vi "InstrumentInteraction ConfigureMeasurementDigits.vi"(6 "contextId":T1, 8 "error in":errorcluster, 9 "timeout (ms)":i32=-1, 10 "Request Data":T3, 11 "gRPC ID":T1) -> (0 "error out":errorcluster, 2 "Response Data":T2, 3 "gRPC ID out":T1)   [LabVIEW 2020, in "Instrument Interaction Client.lvlib"]
uses:
  Instrument Interaction Client.lvlib
  <vilib>/gRPC/LabVIEW gRPC Library/Shared/grpcId.ctl
  RPC Messages/external_driver_wrapper_ConfigureMeasurementDigitsRequest.ctl
  RPC Messages/external_driver_wrapper_ConfigureMeasurementDigitsResponse.ctl
  RPC Messages/external_driver_wrapper_ConfigureMeasurementDigitsResponse_Flat.ctl
  14035477-4c25-4107-8ed5-d0c4ef420ce5.vi
  <vilib>/gRPC/LabVIEW gRPC Library/Shared/TranslateGrpcError.vi
  <vilib>/gRPC/LabVIEW gRPC Library/Shared/Wait On Occurence.vi
  <vilib>/gRPC/LabVIEW gRPC Library/Server API/Server/Get Server DLL Path.vi
  <vilib>/Utility/error.llb/Error Cluster From Error Code.vi
  <vilib>/Utility/error.llb/Simple Error Handler.vi
  <vilib>/gRPC/LabVIEW gRPC Library/grpc-lvsupport-release.lvlib
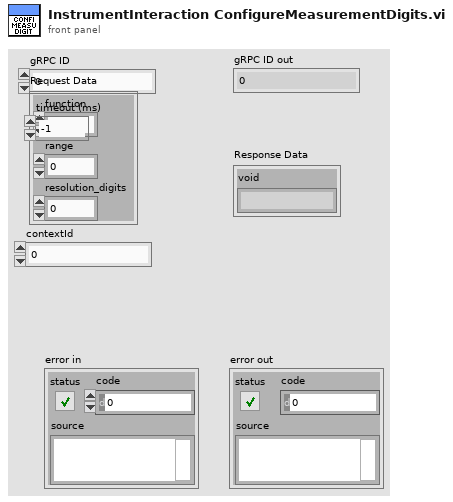
[diagram p1: front panel]
types:
  T1 = typedef "grpc-lvsupport-release.lvlib/grpcId.ctl" = u64
  T2 = typedef "Instrument Interaction Client.lvlib/external_driver_wrapper_ConfigureMeasurementDigitsResponse.ctl" = cluster{"void":string}
  T3 = typedef "Instrument Interaction Client.lvlib/external_driver_wrapper_ConfigureMeasurementDigitsRequest.ctl" = cluster{"function":i32, "range":dbl, "resolution_digits":dbl}
  T4 = typedef "Instrument Interaction Client.lvlib/external_driver_wrapper_ConfigureMeasurementDigitsResponse_Flat.ctl" = cluster{"void":string}
  T5 = typedef "Instrument Interaction Client.lvlib/external_driver_wrapper_ConfigureMeasurementDigitsRequest_Flat.ctl" = cluster{"function":i32, "range":dbl, "resolution_digits":dbl}
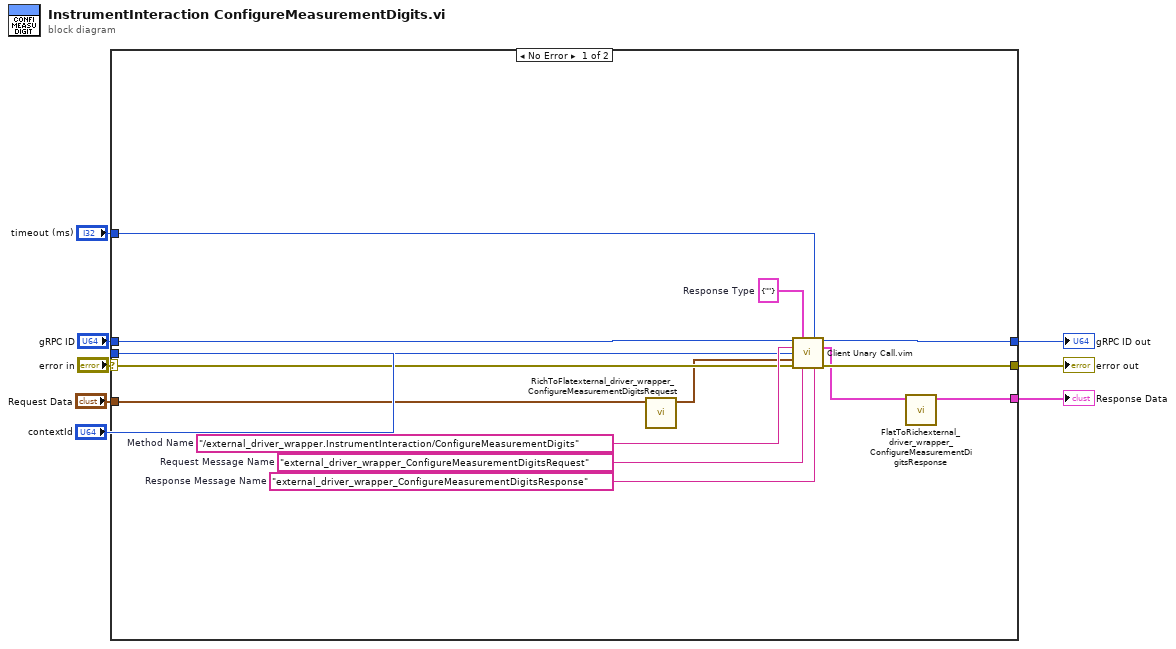
[diagram p0: block diagram]
diagram:
  n1 = case shown="No Error" "error in" {
    selector: "error in" -> [w18 w23]
    tunnel: [w17 w23] -> w7
    tunnel: "gRPC ID" -> [w16 w24]
    tunnel: [w15 w24] -> w5
    tunnel: "Request Data" -> [w12 _]
    tunnel: [w9 _] -> w3
    tunnel: "timeout (ms)" -> [w14 _]
    tunnel: "contextId" -> [w13 _]
    frame No Error {
      w19 = "external_driver_wrapper_ConfigureMeasurementDigitsResponse"  # Response Message Name
      w20 = "external_driver_wrapper_ConfigureMeasurementDigitsRequest"  # Request Message Name
      w21 = T4 {"void"=""}  # Response Type
      w22 = "/external_driver_wrapper.InstrumentInteraction/ConfigureMeasurementDigits"  # Method Name
      n2 = call "RichToFlatexternal_driver_wrapper_ConfigureMeasurementDigitsRequest.vi"("InputCluster"=w12) -> ("OutputCluster"=w11:T5)  [unwired: 10 in]
      n3 = call "Client Unary Call.vim"("ClientID in"=w16, "Response Type"=w21, "timeout (ms)"=w14, "Method Name"=w22, "contextId"=w13, "Request Data"=w11, "error in"=w18, "Request Message Name"=w20, "Response Message Name"=w19) -> ("ClientID out"=w15:u64, "Response Data"=w10:T4, "error out"=w17:errorcluster)  [unwired: 4 in]
      n4 = call "FlatToRichexternal_driver_wrapper_ConfigureMeasurementDigitsResponse.vi"("InputCluster"=w10) -> ("OutputCluster"=w9:T2)  [unwired: 10 in]
    }
    frame Error {
    }
  }
  "error out" <- w7
  "gRPC ID out" <- w5
  "Response Data" <- w3
